vi "lockin - Set REF phase equals zero.vi"(8 "error in (no error)":errorcluster, 11 "Lockin.DAQ out":refnum<class "Instrument.DAQ.lvclass">) -> (0 "error out":errorcluster, 3 "Lockin.DAQ":refnum<class "Instrument.DAQ.lvclass">)   [LabVIEW 2019, in "Instrument.DAQ.lvclass"]
uses:
  Instrument.DAQ.lvclass
  Instrument.DAQ.lvclass/Instrument.DAQ.ctl
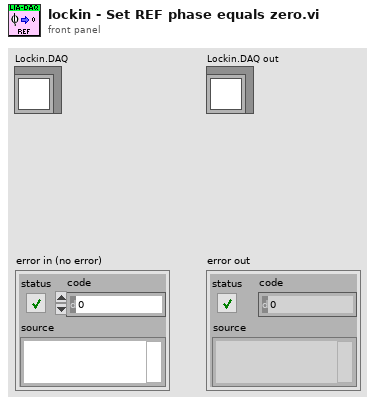
[diagram p1: front panel]
types:
  T1 = typedef "Instrument.DAQ.lvclass/REF-cluster.ctl" = T2[]
  T2 = typedef "Instrument UI.Lockin.lvclass/REF Channel--Cluster.ctl" = cluster{"Enable?":bool, "Channel":i32, "Frequency":dbl, "Phase":dbl, "TC":dbl, "Roll-Off":i32}
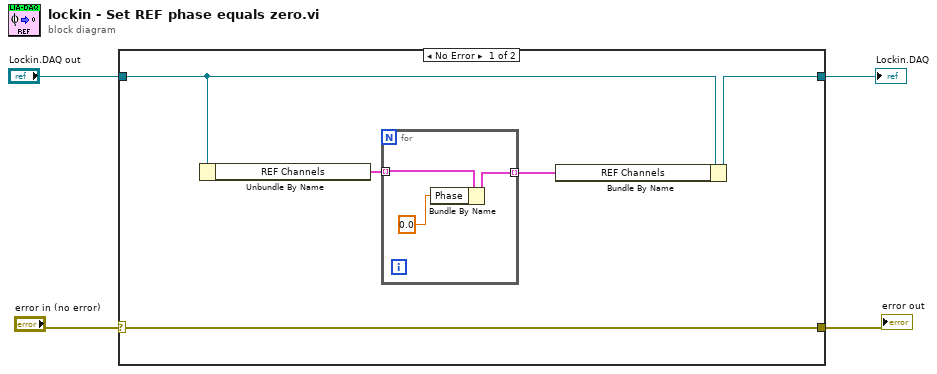
[diagram p0: block diagram]
diagram:
  n1 = case shown="No Error" "error in (no error)" {
    selector: "error in (no error)" -> [w8 w14]
    tunnel: "Lockin.DAQ out" -> [w7 w13]
    tunnel: [w6 w13] -> w3
    tunnel: [w8 w14] -> w1
    frame No Error {
      n2 = Unbundle By Name(w7) -> ("REF Channels"=w9:T1)
      n3 = for {
        tunnel: w9 -> [w12] mode=indexing
        tunnel: [w10] -> w5 mode=indexing
        n4 = Bundle By Name(cluster=w12, "Phase"=0.0) -> (w10:T2)
      }
      n5 = Bundle By Name(cluster=w7, "REF Channels"=w5) -> (w6:refnum<class "Instrument.DAQ.lvclass">)
    }
    frame Error {
    }
  }
  "Lockin.DAQ" <- w3
  "error out" <- w1
